vi "Athletics String Filter.vi"(6 "Answer":T1, 10 "Match String":string, 11 "Classfy In":T2[](array[typedef])) -> (3 "Classfy Out":T2[](array[typedef]))   [LabVIEW 2018]
uses:
  Data Def/Classify.ctl
  Data Def/Answer.ctl
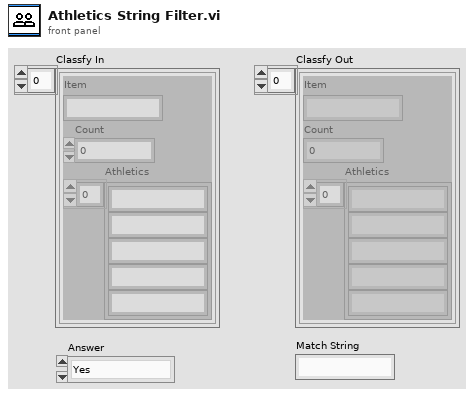
[diagram p1: front panel]
types:
  T1 = typedef "Answer.ctl" = enum16{"Yes", "No", "I don't Know"}
  T2 = typedef "Classify.ctl" = cluster{"Item":string, "Count":i32, "Athletics":string[]}
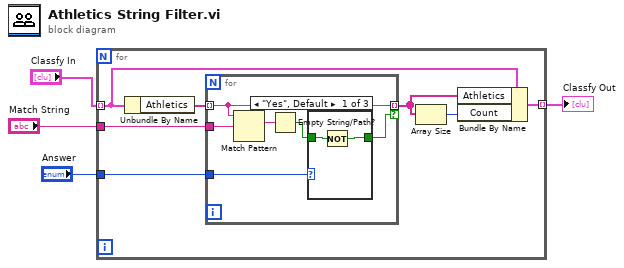
[diagram p0: block diagram]
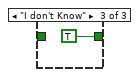
[diagram p3: hidden frame]
diagram:
  n1 = for {
    tunnel: "Classfy In" -> [w8] mode=indexing
    tunnel: "Match String" -> [w10]
    tunnel: "Answer" -> [w9]
    tunnel: [w5] -> w1 mode=indexing
    n2 = Unbundle By Name(w8) -> ("Athletics"=w11:string[])
    n3 = for {
      tunnel: w11 -> [w15] mode=indexing
      tunnel: w10 -> [w17]
      tunnel: w9 -> [w14]
      tunnel: [w15] -> w7 mode=indexing if=w13
      n4 = Match Pattern(string=w15, regular expression=w17) -> (match substring=w16:string)  [unwired: 1 in, 3 out]
      n5 = Empty String/Path?(string/path=w16) -> (empty?=w12:bool)
      n6 = case shown="\"Yes\", Default" w14 {
        tunnel: [w18 w20 TRUE] -> w13
        tunnel: w12 -> [w19 w20 _]
        frame "Yes", Default {
          n7 = Not(x=w19) -> (.not. x?=w18:bool)
        }
        frame "No" {
        }
        frame "I don't Know" {
        }
      }
    }
    n8 = Array Size(array=w7) -> (size(s)=w6:i32)
    n9 = Bundle By Name(cluster=w8, "Athletics"=w7, "Count"=w6) -> (w5:T2)
  }
  "Classfy Out" <- w1
